vi "Add-client.vi"(6 "Client type":T1=enum."Server", 8 "error in (no error)":errorcluster, 9 "Client ID":i32, 10 "Client channel":refnum<queue>, 11 "ModComm in":T2) -> (0 "error out":errorcluster, 3 "ModComm out":T2)   [LabVIEW 2013, in "SLMServer.lvlib" / "SLMServer.lvclass"]
uses:
  SLMServer.lvclass
  Object-reference.ctl
  Supported-module-types.ctl
  SA-SLMAPI/Sources/Message.lvclass
  SLMServer.lvclass/SLMServer.ctl
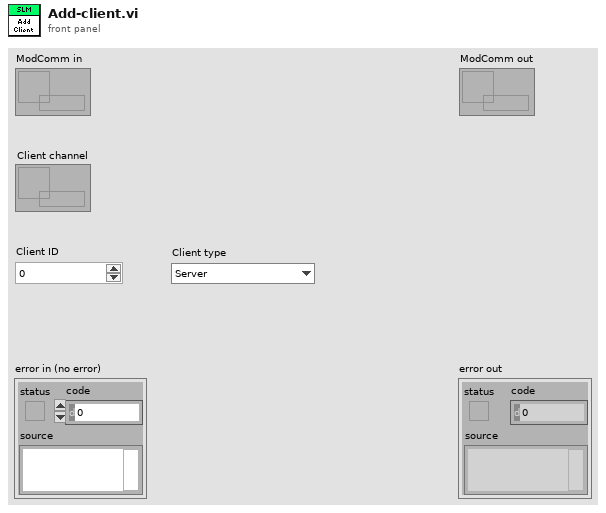
[diagram p1: front panel]
types:
  T1 = typedef "SLMServer.lvlib/SLMServer.lvclass/Supported-module-types.ctl" = enum16{"SLMControl", "PowderDeposition", "CameraVision", "Server", "All", "StrategyParser", "MaterialCharacterization", "StatusMonitor", "SLMSimulation", "LaserCharacterization"}
  T2 = typedef "SLMServer.lvlib/SLMServer.lvclass/Object-reference.ctl" = refnum<data-value>
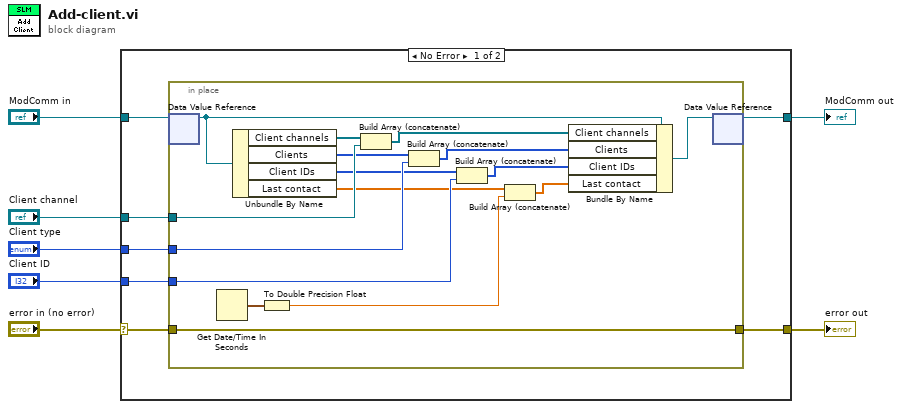
[diagram p0: block diagram]
diagram:
  n1 = case shown="No Error" "error in (no error)" {
    selector: "error in (no error)" -> [w13 w32]
    tunnel: [w8 w32] -> w6
    tunnel: [w9 w31] -> w4
    tunnel: "ModComm in" -> [w14 w31]
    tunnel: "Client channel" -> [w12 _]
    tunnel: "Client type" -> [w11 _]
    tunnel: "Client ID" -> [w10 _]
    frame No Error {
      n2 = in-place {
        in-place-border: w13 -> [w28]
        in-place-border: w12 -> [w26]
        in-place-border: w11 -> [w24]
        in-place-border: w10 -> [w22]
        in-place-border: [w28] -> w8
        n3 = in-place-dvr #1(w14) -> (w30:refnum<class "SLMServer.lvclass">)  [unwired: 1 out]
        n4 = Get Date/Time In Seconds() -> (seconds since 1Jan1904=w20:timestamp)
        n5 = Unbundle By Name(w30) -> ("Client channels"=w27:refnum<queue>[], "Clients"=w25:T1[], "Client IDs"=w23:i32[], "Last contact"=w21:dbl[])
        n6 = To Double Precision Float(number=w20) -> (double precision float=w19:dbl)
        n7 = Build Array (concatenate)(w27, w26) -> (w15:refnum<queue>[])
        n8 = Build Array (concatenate)(w25, w24) -> (w16:T1[])
        n9 = Build Array (concatenate)(w23, w22) -> (w17:i32[])
        n10 = Build Array (concatenate)(w21, w19) -> (w18:dbl[])
        n11 = Bundle By Name(cluster=w30, "Client channels"=w15, "Clients"=w16, "Client IDs"=w17, "Last contact"=w18) -> (w29:refnum<class "SLMServer.lvclass">)
        n12 = in-place-dvr #1(w29) -> (w9:T2)  [unwired: 1 out]
      }
    }
    frame Error {
    }
  }
  "error out" <- w6
  "ModComm out" <- w4
